vi "Last_modified_date.vi"(0 "Update Now":bool) -> (1 "RevisionString":string, 2 "BasesvnRevision":u32)   [LabVIEW 2012]
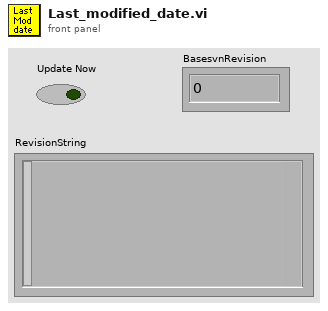
[diagram p1: front panel]
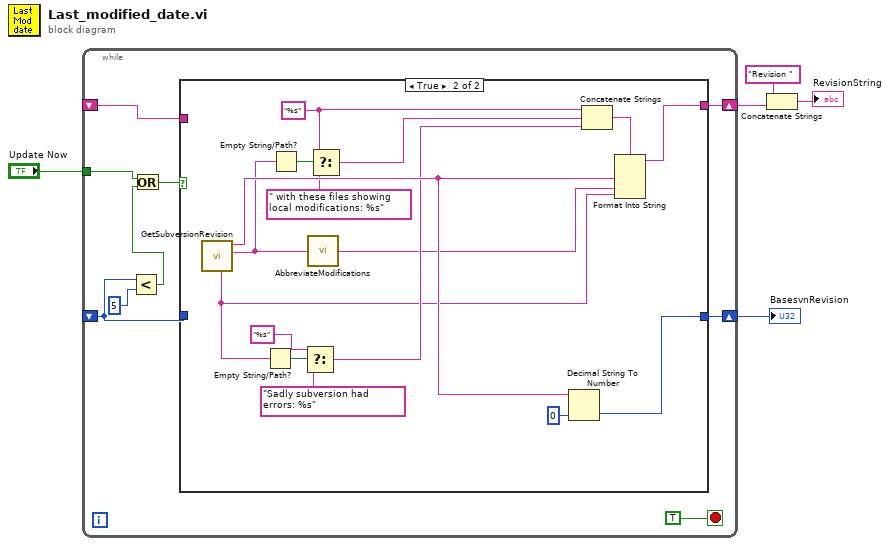
[diagram p0: block diagram]
diagram:
  n1 = while {
    shift-right: [w14] -> w5
    shift-left: _ -> [w13]
    shift-right: [w11] -> w4
    shift-left: _ -> [w8]
    tunnel: "Update Now" -> [w9]
    stop <- TRUE stop-if-true
    n2 = Less?(x=w8, y=u32 5) -> (x < y?=w6:bool)
    n3 = Or(x=w9, y=w6) -> (x .or. y?=w10:bool)
    n4 = case shown="True" w10 {
      tunnel: [w16 w30] -> w14
      tunnel: w13 -> [w16 _]
      tunnel: [w15 w32] -> w11
      tunnel: w8 -> [w15 _]
      frame False {
      }
      frame True {
        w26 = "%s" ("format string")
        n5 = call "GetSubversionRevision.vi"() -> ("LocalModifications"=w19:string, "OverallRevision"=w31:string, "standard error"=w20:string)  [unwired: 6 in, 3 out]
        n6 = Empty String/Path?(string/path=w20) -> (empty?=w23:bool)
        n7 = Empty String/Path?(string/path=w19) -> (empty?=w29:bool)
        n8 = Select(t="%s" ("format string"), s=w23, f="Sadly subversion had errors: %s" ("format string")) -> (s? t:f=w21:string)
        n9 = call "AbbreviateModifications.vi"("svnString"=w19) -> ("VInames"=w18:string)  [unwired: 4 in]
        n10 = Select(t=w26, s=w29, f=" with these files showing local modifications: %s" ("format string")) -> (s? t:f=w27:string)
        n11 = Decimal String To Number(string=w31, default (0L)=u32 0 ("default (0 I32)")) -> (number=w32:u32)  [unwired: 1 in, 1 out]
        n12 = Concatenate Strings(w26, w27, w21) -> (w25:string)
        n13 = Format Into String(format string=w25, w31, w18, w20) -> (resulting string=w30:string)  [unwired: 2 in, 1 out]
      }
    }
  }
  "BasesvnRevision" <- w4
  n14 = Concatenate Strings("Revision " ("string"), w5) -> (→"RevisionString":string)
